vi "tagDB_Value_Template_Ref.vi"(6 "Add wih NonExist?":bool, 8 "error in (no error)":errorcluster, 9 "Type":refnum<vi>, 10 "name":string, 11 "DB Ref":T1) -> (0 "error out":errorcluster, 2 "value":refnum<vi>, 3 "DB Ref(dup)":T1)   [LabVIEW 2014, in "TagDB(dev).lvlib"]
doc: "[Covers: REQ_TAGDB_TEMPLATE_VALUE_REF]"
uses:
  tagDB_Def.ctl
  Error/_[error50001]Can't Found Value.vi
  Private/_Cast TagDB Ref to DVR.vi
  _global/URL/TRIM-BOTH-SPACE.vi
  Error/_[error50000]Invalid DB REF.vi
  TagDB(dev).lvlib
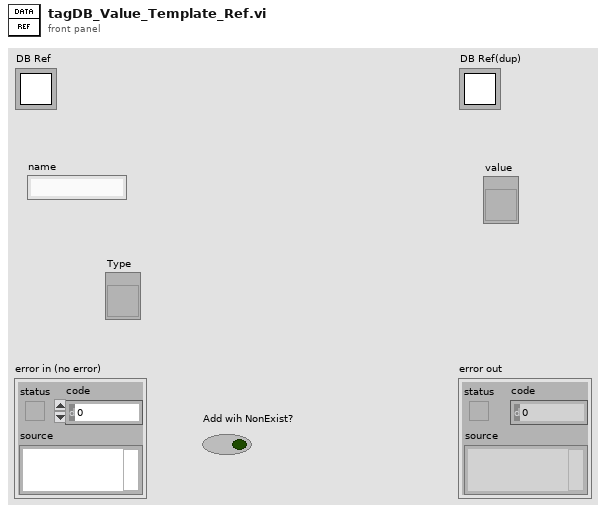
[diagram p1: front panel]
types:
  T1 = typedef "TagDB(dev).lvlib/tagDB_Def.ctl" = refnum<k1>
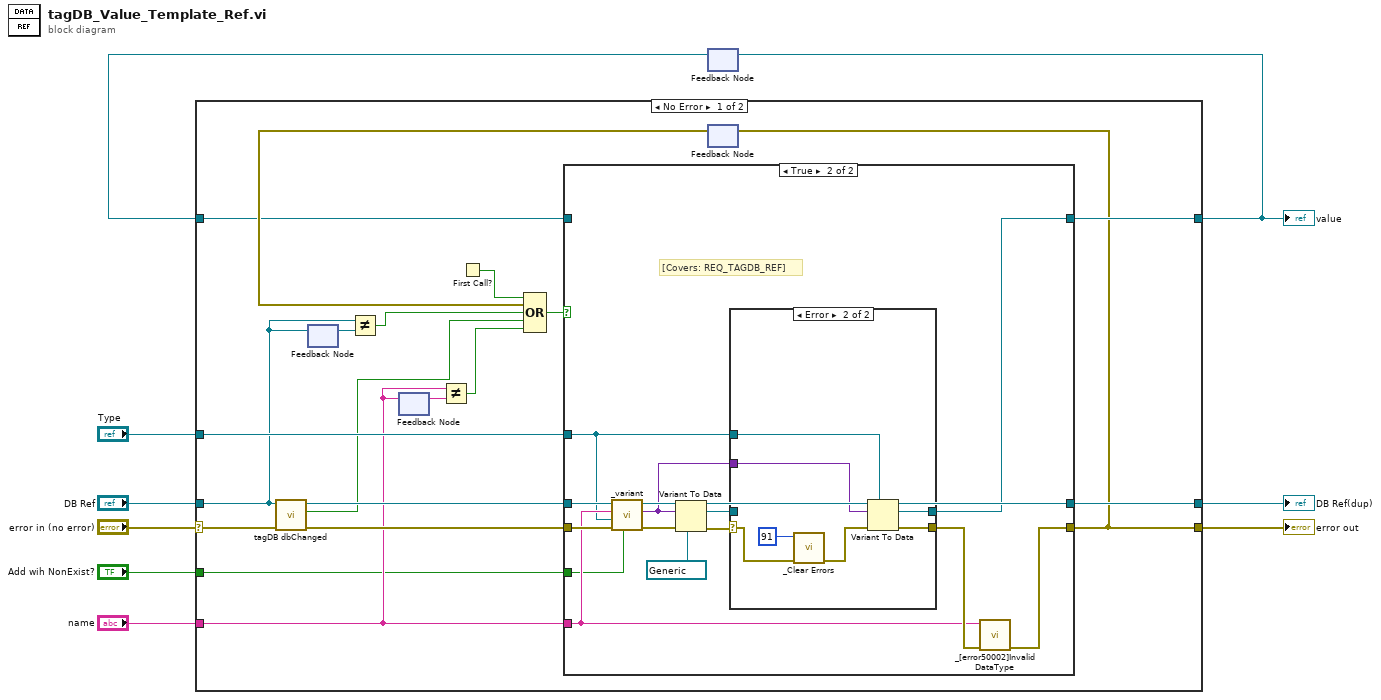
[diagram p0: block diagram]
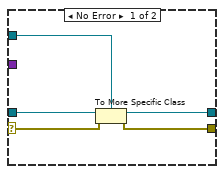
[diagram p3: hidden frame]
diagram:
  n1 = feedback #1() -> (w2:refnum<vi>)  [unwired: 1 in]
  n2 = case shown="No Error" "error in (no error)" {
    selector: "error in (no error)" -> [w23 w60]
    tunnel: [w14 w60] -> w8
    tunnel: [w28 w59] -> w6
    tunnel: "DB Ref" -> [w15 w59]
    tunnel: "name" -> [w16 _]
    tunnel: "Type" -> [w26 _]
    tunnel: [w27 w58] -> w3
    tunnel: w2 -> [w11 w58]
    tunnel: "Add wih NonExist?" -> [w10 _]
    frame No Error {
      n3 = call "tagDB dbChanged.vi"("error in (no error)"=w23, "DB Ref"=w15) -> ("error in (no error) (dup)"=w24:errorcluster, "changed?"=w17:bool, "DB Ref (dup)"=w25:T1)  [unwired: 7 in]
      n4 = feedback #2() -> (w21:T1)  [unwired: 1 in]
      n5 = feedback-in #2(w15) -> ()
      n6 = Not Equal?(x=w15, y=w21) -> (x != y?=w19:bool)
      n7 = feedback #3() -> (w20:string)  [unwired: 1 in]
      n8 = feedback-in #3(w16) -> ()
      n9 = Not Equal?(x=w16, y=w20) -> (x != y?=w18:bool)
      n10 = First Call?() -> (First Call?: T/F=w22:bool)
      n11 = feedback #4() -> (w13:errorcluster)  [unwired: 1 in]
      n12 = Compound Arithmetic op=OR(w22, w13, w19, w17, w18) -> (w12:bool)
      n13 = case shown="True" w12 {
        tunnel: [w31 w44] -> w28
        tunnel: [w29 w38] -> w27
        tunnel: w26 -> [_ w32]
        tunnel: w25 -> [w31 w37]
        tunnel: w24 -> [w30 w36]
        tunnel: w16 -> [_ w35]
        tunnel: [w30 w34] -> w14
        tunnel: w11 -> [w29 _]
        tunnel: w10 -> [_ w33]
        frame False {
        }
        frame True {
          # "[Covers: REQ_TAGDB_REF]"
          n14 = call "_variant.vi"("Add wih NonExist?"=w33, "error in (no error)"=w36, "default value (empty variant)"=w32, "name"=w35, "DB Ref"=w37) -> ("error out"=w45:errorcluster, "value"=w43:variant, "DB Ref (dup)"=w44:T1)  [unwired: 4 in]
          n15 = Variant To Data(error in=w45, type=refnum<vi> refnum ("value"), Variant=w43) -> (data=w39:refnum<vi>, error out=w40:errorcluster)
          n16 = case shown="Error" w40 {
            selector: w40 -> [w48 w57]
            tunnel: [w49 w51] -> w38
            tunnel: [w47 w54] -> w42
            tunnel: w32 -> [w46 w52]
            tunnel: w39 -> [w50 _]
            tunnel: w43 -> [_ w53]
            frame No Error {
              n17 = To More Specific Class(target class=w46, reference=w50, error in=w48) -> (specific class reference=w49:refnum<vi>, error out=w47:errorcluster)
            }
            frame Error {
              n18 = call "_Clear Errors.vi"("error in (no error)"=w57, "specific error code to clear (0: all)"=91) -> ("error out"=w55:errorcluster)  [unwired: 4 in, 1 out]
              n19 = Variant To Data(error in=w55, type=w52, Variant=w53) -> (data=w51:refnum<vi>, error out=w54:errorcluster)
            }
          }
          n20 = call "_[error50002]Invalid DataType.vi"("error in (no error)"=w42, "string"=w35) -> ("error out"=w34:errorcluster)  [unwired: 9 in]
        }
      }
      n21 = feedback-in #4(w14) -> ()
    }
    frame Error {
    }
  }
  "error out" <- w8
  "DB Ref(dup)" <- w6
  "value" <- w3
  n22 = feedback-in #1(w3) -> ()
